vi "measure_voltage_new.vi"(9 "rate":dbl=100.0, 11 "number of samples":i32=100) -> (1 "data":dynamicdata(graph), 3 "F-format string":string)   [LabVIEW 2017]
uses:
  <vilib>/Analysis/baseanly.llb/Mean (DBL).vi
  <vilib>/Analysis/NI_AALBase.lvlib
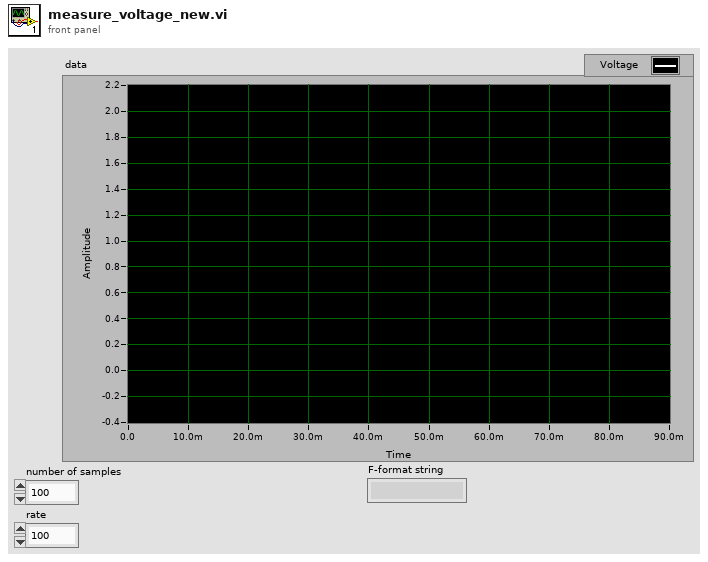
[diagram p1: front panel]
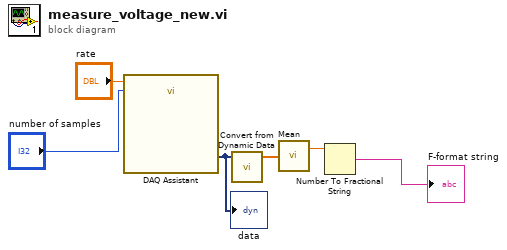
[diagram p0: block diagram]
diagram:
  n1 = call "DAQ Assistant"("rate"="rate", "number of samples"="number of samples") -> ("data"=w4:dynamicdata)  [unwired: 15 in, 2 out]
  "data" <- w4
  n2 = call "Convert from Dynamic Data"("Dynamic Data Type"=w4) -> ("Array"=w3:dbl[])  [unwired: 3 in]
  n3 = call-poly <vilib>:"Mean.vi"("X"=w3) -> ("mean"=w2:dbl)  [unwired: 1 out]
  n4 = Number To Fractional String(number=w2) -> (F-format string=→"F-format string":string)  [unwired: 3 in]
